vi "Core Init.vi"(4 "2nd Panel":refnum<vi>, 6 "1st Panel":refnum<vi>, 8 "error in (no error)":errorcluster, 10 "Splitter ref":refnum<vi>, 11 "DualScreen in":refnum<class "DualScreen.lvclass">) -> (0 "error out":errorcluster, 3 "DualScreen out":refnum<class "DualScreen.lvclass">)   [LabVIEW 2020, in "DualScreen.lvlib" / "DualScreen.lvclass"]
uses:
  DualScreen.lvclass
  D:/Projets/STEP AT/Bahamut/support/UI_Actor.lvlibp/UI_Actor/UI_Actor.lvclass
  DualScreen.lvclass/DualScreen.ctl
  support/UI_Actor.lvlibp/UI_Actor/Read Name.vi
  support/UI_Actor.lvlibp/UI_Actor/UI_Actor.lvclass
  D:/Projets/STEP AT/Bahamut/D&Cs/D&C_SchemaBase/D&C_SchemaBase/D&C_SchemaBase.lvclass
  D:/Projets/STEP AT/Bahamut/support/Actor Framework.lvlibp/1abvi3w/vi.lib/ActorFramework/Actor/Actor.lvclass
  D:/Projets/STEP AT/Bahamut/D&Cs/DualScreen/DualScreen/DualScreen.lvclass
  support/UI_Actor.lvlibp/UI_Actor Messages/UI_ShowIn_Subpanel Msg/UI_ShowIn_Subpanel Msg.lvclass
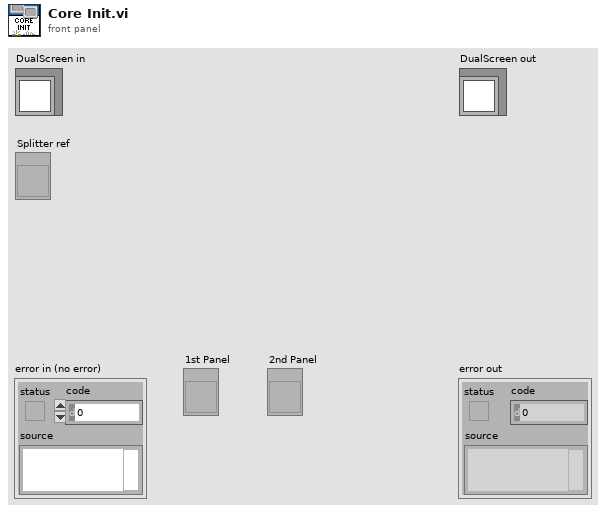
[diagram p1: front panel]
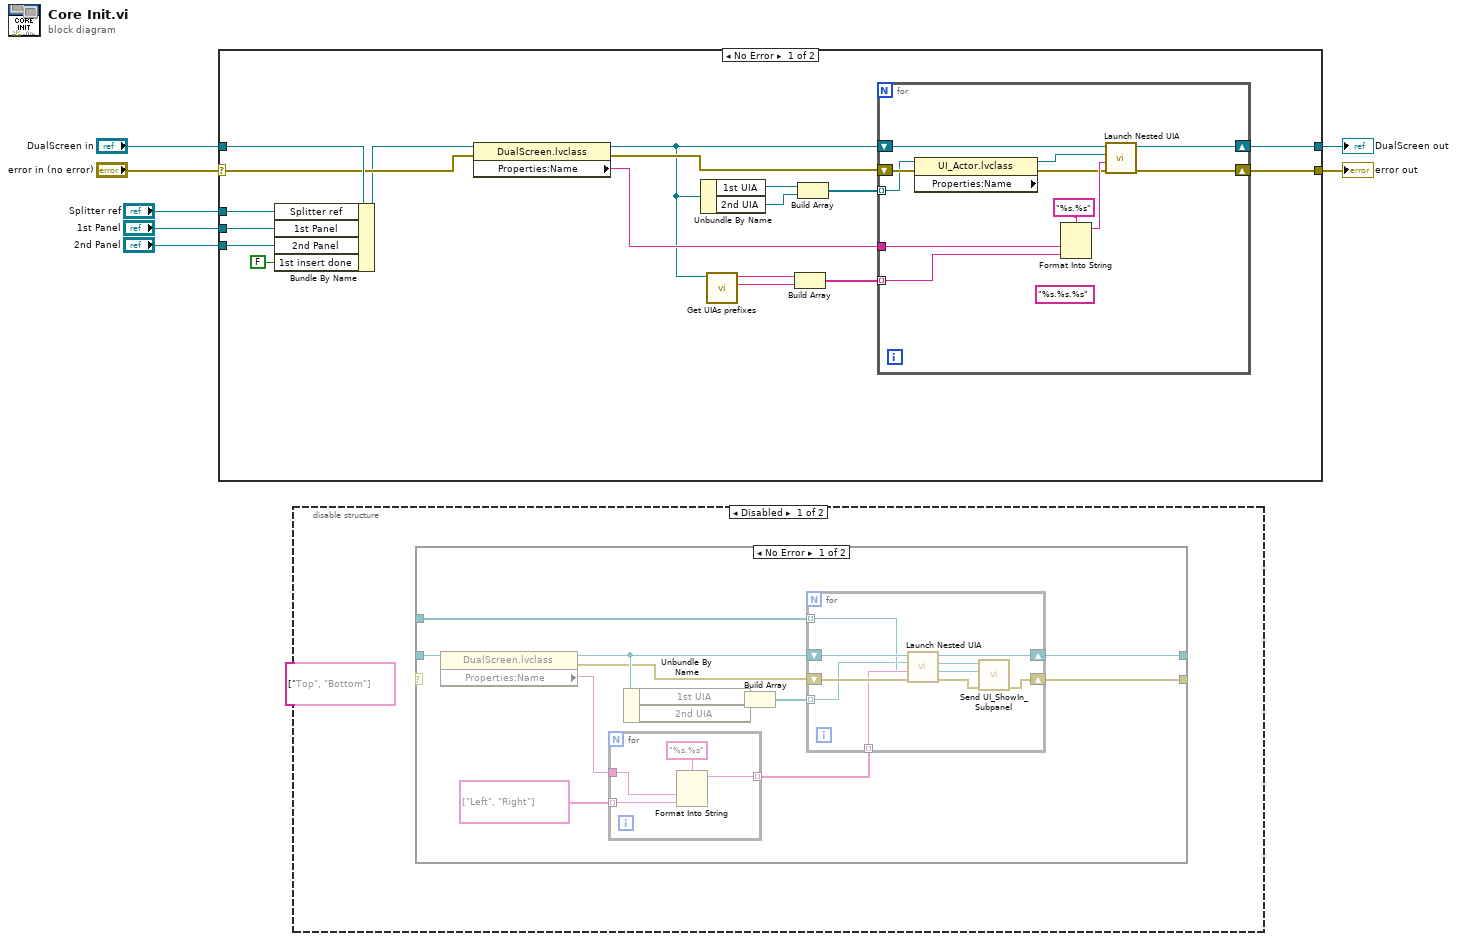
[diagram p0: block diagram]
diagram:
  n1 = case shown="No Error" "error in (no error)" {
    selector: "error in (no error)" -> [w21 w38]
    tunnel: [w13 w38] -> w6
    tunnel: [w15 w37] -> w4
    tunnel: "DualScreen in" -> [w25 w37]
    tunnel: "2nd Panel" -> [w24 _]
    tunnel: "1st Panel" -> [w23 _]
    tunnel: "Splitter ref" -> [w22 _]
    frame No Error {
      n2 = Bundle By Name(cluster=w25, "Splitter ref"=w22, "1st Panel"=w23, "2nd Panel"=w24, "1st insert done"=FALSE) -> (w16:refnum<class "DualScreen.lvclass">)
      n3 = property class="DualScreen.lvclass"(reference=w16, error in=w21) -> (reference out=w12:refnum<class "DualScreen.lvclass">, error out=w17:errorcluster, "Properties:Name"=w14:string)
      n4 = Unbundle By Name(w12) -> ("1st UIA"=w20:refnum<class "UI_Actor.lvclass">, "2nd UIA"=w19:refnum<class "UI_Actor.lvclass">)
      n5 = call-dynamic "Get UIAs prefixes.vi"("DualScreen in"=w12) -> ("2nd UIA prefix"=w10:string, "1st UIA prefix"=w11:string)  [unwired: 9 in]
      n6 = Build Array(w11, w10) -> (w9:string[])
      n7 = Build Array(w20, w19) -> (w18:refnum<class "UI_Actor.lvclass">[])
      n8 = for {
        shift-right: [w35] -> w15
        shift-left: w12 -> [w36]
        shift-right: [w27] -> w13
        shift-left: w17 -> [w31]
        tunnel: w18 -> [w29] mode=indexing
        tunnel: w14 -> [w33]
        tunnel: w9 -> [w26] mode=indexing
        (unwired) "%s.%s.%s" ("format string")
        n9 = property class="UI_Actor.lvclass" props=["Properties:Name"](reference=w29, error in=w31) -> (reference out=w30:refnum<class "UI_Actor.lvclass">, error out=w28:errorcluster)  [unwired: 1 out]
        n10 = Format Into String(format string="%s.%s", w33, w26) -> (resulting string=w32:string)  [unwired: 2 in, 1 out]
        n11 = call "Launch Nested UIA.vi"("error in (no error)"=w28, "Name"=w32, "UI_Actor"=w30, "Caller UIA in"=w36) -> ("error out"=w27:errorcluster, "Caller UIA out"=w35:refnum<class "DualScreen.lvclass">)  [unwired: 5 in, 1 out]
      }
    }
    frame Error {
    }
  }
  "error out" <- w6
  "DualScreen out" <- w4
  n12 = disable-structure shown="Disabled" {
    frame Disabled {
      (unwired) string[] ["Top", "Bottom"]
      n13 = case shown="No Error" {
        selector: _ -> [_ w65]
        tunnel: [w49 w65] -> _
        tunnel: [w48 w64] -> _
        tunnel: _ -> [w43 w64]
        tunnel: _ -> [w50 _]
        frame No Error {
          n14 = property class="DualScreen.lvclass"(reference=w43) -> (reference out=w44:refnum<class "DualScreen.lvclass">, error out=w41:errorcluster, "Properties:Name"=w42:string)  [unwired: 1 in]
          n15 = for {
            tunnel: w42 -> [w52]
            tunnel: string[] ["Left", "Right"] -> [w51] mode=indexing
            tunnel: [w54] -> w39 mode=indexing
            n16 = Format Into String(format string="%s.%s", w52, w51) -> (resulting string=w54:string)  [unwired: 2 in, 1 out]
          }
          n17 = Unbundle By Name(w44) -> ("1st UIA"=w47:refnum<class "UI_Actor.lvclass">, "2nd UIA"=w46:refnum<class "UI_Actor.lvclass">)
          n18 = Build Array(w47, w46) -> (w45:refnum<class "UI_Actor.lvclass">[])
          n19 = for {
            shift-right: [w60] -> w48
            shift-left: w44 -> [w63]
            shift-right: [w56] -> w49
            shift-left: w41 -> [w62]
            tunnel: w39 -> [w61] mode=indexing
            tunnel: w50 -> [w58] mode=indexing
            tunnel: w45 -> [w55] mode=indexing
            n20 = call "Launch Nested UIA.vi"("error in (no error)"=w62, "Name"=w61, "UI_Actor"=w55, "Caller UIA in"=w63) -> ("error out"=w57:errorcluster, "Nested Actor's Enqueuer"=w59:refnum<class "Message Enqueuer.lvclass">, "Caller UIA out"=w60:refnum<class "DualScreen.lvclass">)  [unwired: 5 in]
            n21 = call "Send UI_ShowIn_Subpanel.vi"("error in (no error)"=w57, "Sub Panel"=w58, "Message Enqueuer"=w59) -> ("error out"=w56:errorcluster)  [unwired: 7 in, 1 out]
          }
        }
        frame Error {
        }
      }
    }
    frame Enabled {
    }
  }
